vi "Create RYB Traditional Color Scale Array.vi"() -> (2 "Must Include":u32[](array[colorbox])=[16711680, 16733001, 16744448, 16760576, 16776960, 8442906, 43571, 1410150, 2777241, 5582989, 8388736, 12517441, 16711680], 3 "RYB Array":u32[](array[colorbox]))   [LabVIEW 2015, in "ColorSelector.lvclass"]
doc: "This VI creates a Red-Yellow-Blue (RYB) Color Scale Array that aligns with the more traditional paint colors one is taught in grade school. This scale includes:\n\n\nFF0000 Red Primary \nFF5349 Vermillion Tertiary\nFF8000 Orange Secondary\nFFBF00 Amber Tertiary\nFFFF00 Yellow Primary\n80D41A Chartreuse Tertiary\n00AA33 Green Secondary\n158466 Teal Tertiary\n2A6099 Blue Primary\n55308D Violet Tertiary\n800080 Purple Secondary\nBF0041 Magenta Tertiary\n<b> </b> <b> </b>\n©2017 Q Software Innovations, LLC (QSI)\nwritten by Quentin Alldredge\nproduced in LabVIEW 2015\n\nsupport@qsoftwareinnovations.com\nwww.qsoftwareinnovations.com\n\nAll rights reserved.\n\nRedistribution and use in source and binary forms, with or without modification, are permitted provided that the following conditions are met:\n\n * Redistributions of source code must retain the above copyright notice, this list of conditions and the following disclaimer.\n * Redistributions in binary form must reproduce the above copyright notice, this list of conditions and the following disclaimer in the documentation and/or other materials provided with the distribution.\n * Neither the name of Q Software Innovations, LLC. nor the names of its contributors may be used to endorse or promote products derived from this software without specific prior written permission.\n\nTHIS SOFTWARE IS PROVIDED BY THE COPYRIGHT HOLDERS AND CONTRIBUTORS \"AS IS\" AND ANY EXPRESS OR IMPLIED WARRANTIES, INCLUDING, BUT NOT LIMITED TO, THE IMPLIED WARRANTIES OF MERCHANTABILITY AND FITNESS FOR A PARTICULAR PURPOSE ARE DISCLAIMED. IN NO EVENT SHALL THE COPYRIGHT OWNER OR CONTRIBUTORS BE LIABLE FOR ANY DIRECT, INDIRECT, INCIDENTAL, SPECIAL, EXEMPLARY, OR CONSEQUENTIAL DAMAGES (INCLUDING, BUT NOT LIMITED TO, PROCUREMENT OF SUBSTITUTE GOODS OR SERVICES; LOSS OF USE, DATA, OR PROFITS; OR BUSINESS INTERRUPTION) HOWEVER CAUSED AND ON ANY THEORY OF LIABILITY, WHETHER IN CONTRACT, STRICT LIABILITY, OR TORT (INCLUDING NEGLIGENCE OR OTHERWISE) ARISING IN ANY WAY OUT OF THE USE OF THIS SOFTWARE, EVEN IF ADVISED OF THE POSSIBILITY OF SUCH DAMAGE."
uses:
  ColorSelector.lvclass
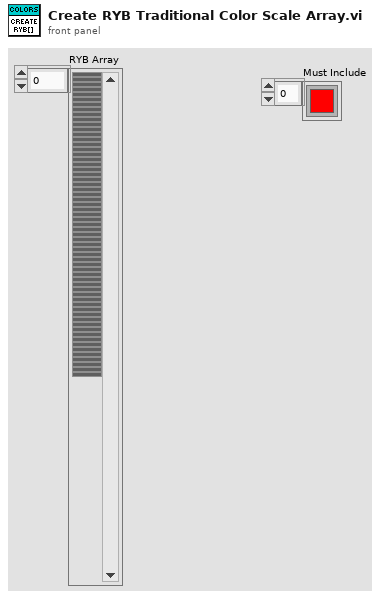
[diagram p1: front panel]
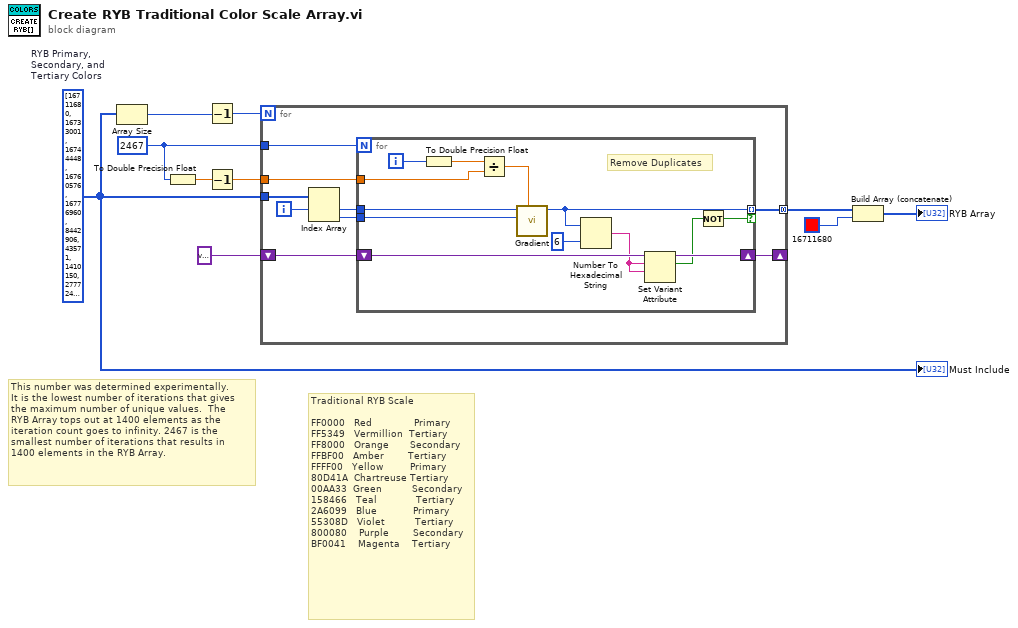
[diagram p0: block diagram]
diagram:
  w2 = 2467
  w7 = u32[] [16711680, 16733001, 16744448, 16760576, 16776960, 8442906, 43571, 1410150, 2777241, 5582989, 8388736, 12517441, 16711680]  # RYB Primary,  Secondary, and  Tertiary Colors
  # "Traditional RYB Scale\n\nFF0000   Red              Primary\t\nFF5349   Vermillion\t Tertiary\nFF8000   Orange\t      Secondary\nFFBF00   Amber        Tertiary\nFFFF00   Yellow         Primary\n80D41A  Chartreuse\tTertiary\n00AA33  Green          Secondary\n158466   Teal             Tertiary\n2A6099   Blue\t           Primary\n55308D   Violet          Tertiary\n800080    Purple\t       Secondary\nBF0041    Magenta\t   Tertiary"
  # "This number was determined experimentally.  \nIt is the lowest number of iterations that gives \nthe maximum number of unique values.  The \nRYB Array tops out at 1400 elements as the \niteration count goes to infinity. 2467 is the \nsmallest number of iterations that results in\n1400 elements in the RYB Array."
  n1 = Array Size(array=w7) -> (size(s)=w6:i32)
  n2 = To Double Precision Float(number=w2) -> (double precision float=w10:dbl)
  n3 = Decrement(x=w6) -> (x-1=w5:i32)
  n4 = Decrement(x=w10) -> (x-1=w9:dbl)
  n5 = for {
    N: w5 -> [_]
    tunnel: w7 -> [w19]
    tunnel: w9 -> [w15]
    tunnel: w2 -> [w14]
    tunnel: [w13] -> w8 mode=concatenating
    shift-right: [w11] -> _
    shift-left: variant -> [w12]
    i -> [w18]
    n6 = Index Array(array=w19, index #1=w18) -> (element #1=w17:u32, element #2=w16:u32)  [unwired: 1 in]
    n7 = for {
      N: w14 -> [_]
      tunnel: [w26] -> w13 mode=indexing if=w21
      tunnel: w17 -> [w31]
      tunnel: w16 -> [w30]
      tunnel: w15 -> [w28]
      shift-right: [w23] -> w11
      shift-left: w12 -> [w24]
      i -> [w32]
      # "Remove Duplicates"
      n8 = To Double Precision Float(number=w32) -> (double precision float=w29:dbl)
      n9 = Divide(x=w29, y=w28) -> (x/y=w27:dbl)
      n10 = call "Gradient.vi"("Percent"=w27, "End Color"=w30, "Start Color"=w31) -> ("Gradient Color"=w26:u32)  [unwired: 8 in]
      n11 = Number To Hexadecimal String(1:i16 6 ("width (-)"), 2:w26) -> (0:w20:string)
      n12 = Set Variant Attribute(Variant=w24, name=w20, value=w20) -> (Variant out=w23:variant, replaced=w22:bool)  [unwired: 1 in, 1 out]
      n13 = Not(x=w22) -> (.not. x?=w21:bool)
    }
  }
  n14 = Build Array (concatenate)(w8, u32 16711680) -> (→"RYB Array":u32[])
  "Must Include" <- w7
